vi "Day3Part2.vi"(11 "Input":string) -> (3 "Result":i64)   [LabVIEW 2024]
uses:
  <vilib>/regexp/Match Regular Expression.xnode
panel:
  out "Array 3":string[](array[string])
  out "Array 2":string[](array[string])
  out "Array":string[](array[string])
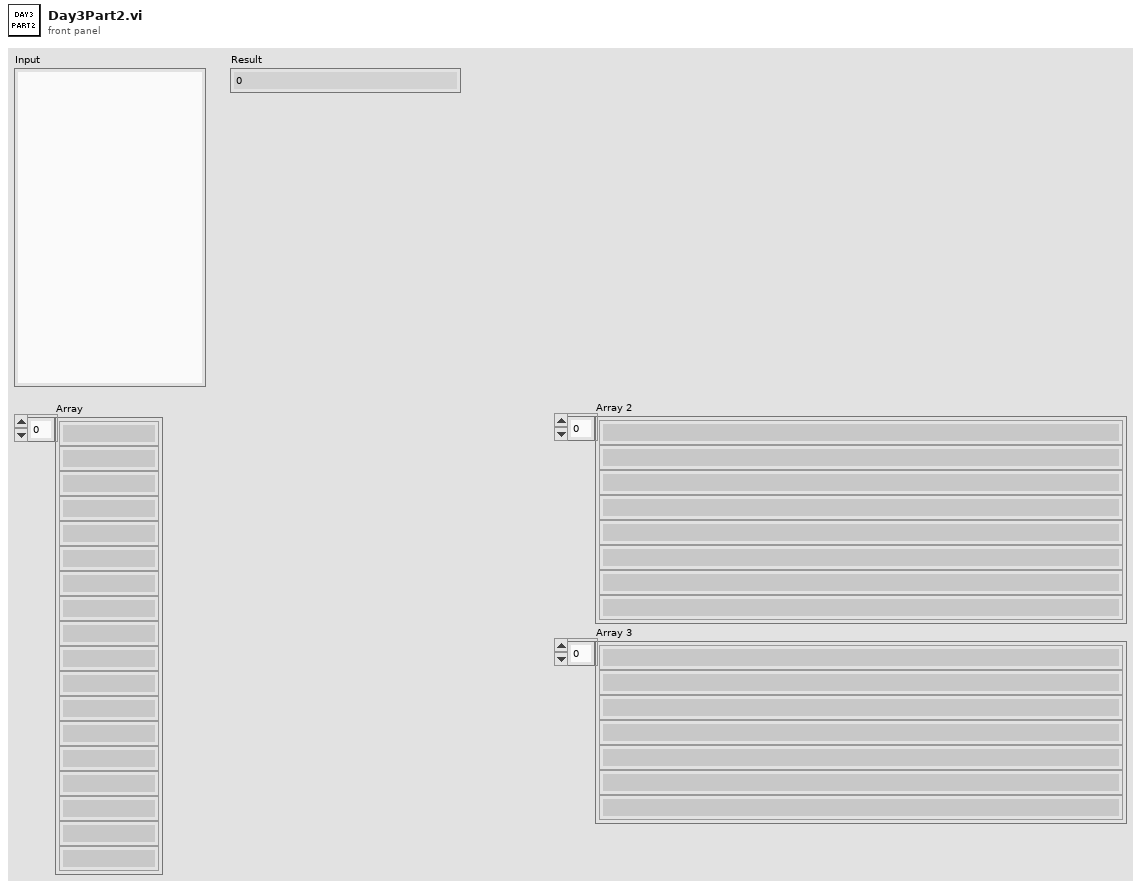
[diagram p1: front panel]
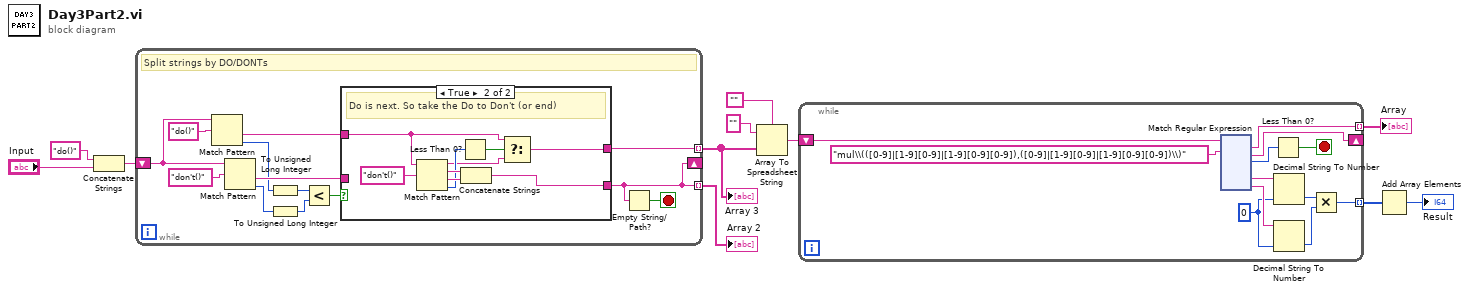
[diagram p0: block diagram]
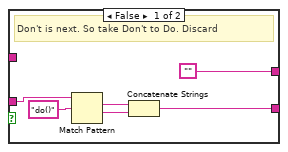
[diagram p2: hidden frame]
diagram:
  n1 = Concatenate Strings("do()" ("string"), "Input") -> (w3:string)
  n2 = while {
    shift-right: [w16] -> _
    shift-left: w3 -> [w20]
    tunnel: [w21] -> w8 mode=indexing
    tunnel: [w16] -> w2 mode=indexing
    stop <- w18 stop-if-true
    # "Split strings by DO/DONTs"
    n3 = Match Pattern(string=w20, regular expression="do()") -> (after substring=w19:string, offset past match=w13:i32)  [unwired: 1 in, 2 out]
    n4 = Match Pattern(string=w20, regular expression="don't()") -> (after substring=w17:string, offset past match=w15:i32)  [unwired: 1 in, 2 out]
    n5 = To Unsigned Long Integer(number=w13) -> (unsigned 32bit integer=w12:u32)
    n6 = To Unsigned Long Integer(number=w15) -> (unsigned 32bit integer=w14:u32)
    n7 = Less?(x=w12, y=w14) -> (x < y?=w22:bool)
    n8 = case shown="True" w22 {
      tunnel: ["" w33] -> w21
      tunnel: w17 -> [w29 _]
      tunnel: w19 -> [_ w34]
      tunnel: [w26 w32] -> w16
      frame False {
        # "Don't is next. So take Don't to Do. Discard"
        n9 = Match Pattern(string=w29, regular expression="do()") -> (match substring=w28:string, after substring=w27:string)  [unwired: 1 in, 2 out]
        n10 = Concatenate Strings(w28, w27) -> (w26:string)
      }
      frame True {
        # "Do is next. So take the Do to Don't (or end)"
        n11 = Match Pattern(string=w34, regular expression="don't()") -> (before substring=w31:string, match substring=w38:string, after substring=w37:string, offset past match=w36:i32)  [unwired: 1 in]
        n12 = Less Than 0?(x=w36) -> (x < 0?=w35:bool)
        n13 = Concatenate Strings(w38, w37) -> (w32:string)
        n14 = Select(t=w34, s=w35, f=w31) -> (s? t:f=w33:string)
      }
    }
    n15 = Empty String/Path?(string/path=w16) -> (empty?=w18:bool)
  }
  "Array 2" <- w2
  "Array 3" <- w8
  n16 = Array To Spreadsheet String(delimiter (Tab)="", array=w8, 3:"" ("format string")) -> (spreadsheet string=w5:string)
  n17 = while {
    shift-right: [w49] -> _
    shift-left: w5 -> [w51]
    tunnel: [w44] -> w11 mode=indexing
    tunnel: [w42] -> w9 mode=indexing
    stop <- w40 stop-if-true
    w43 = i64 0 ("default (0 I32)")
    n18 = xnode "Match Regular Expression"("input string"=w51, "regular expression"="mul\\(([0-9]|[1-9][0-9]|[1-9][0-9][0-9]),([0-9]|[1-9][0-9]|[1-9][0-9][0-9])\\)") -> ("whole match"=w42:string, "after match"=w49:string, "offset past match"=w41:i32, "submatch 1"=w48:string, "submatch 2"=w47:string)  [unwired: 4 in, 2 out]
    n19 = Less Than 0?(x=w41) -> (x < 0?=w40:bool)
    n20 = Decimal String To Number(string=w48, default (0L)=w43) -> (number=w46:i64)  [unwired: 1 in, 1 out]
    n21 = Decimal String To Number(string=w47, default (0L)=w43) -> (number=w45:i64)  [unwired: 1 in, 1 out]
    n22 = Multiply(x=w46, y=w45) -> (x*y=w44:i64)
  }
  "Array" <- w9
  n23 = Add Array Elements(numeric array=w11) -> (sum=→"Result":i64)
